vi "Project VIs.vi"(8 "Error In":errorcluster, 11 "Proejct Target App In":refnum<vi>) -> (0 "Error Out":errorcluster, 2 "VIs":T1[](array[typedef]), 3 "Project Target App Out":refnum<vi>)   [LabVIEW 2017, in "Bookmark Manager.lvlib"]
uses:
  Bookmark Manager.lvlib
  Controls/VI Information.ctl
  Controls/Application Information.ctl
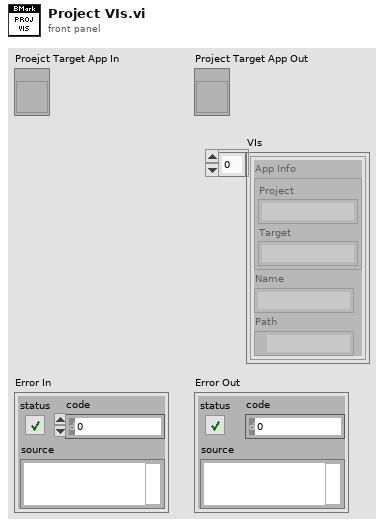
[diagram p1: front panel]
types:
  T1 = typedef "Bookmark Manager.lvlib/VI Information.ctl" = cluster{"App Info":T2, "Name":string, "Path":path}
  T2 = typedef "Bookmark Manager.lvlib/Application Information.ctl" = cluster{"Project":string, "Target":string}
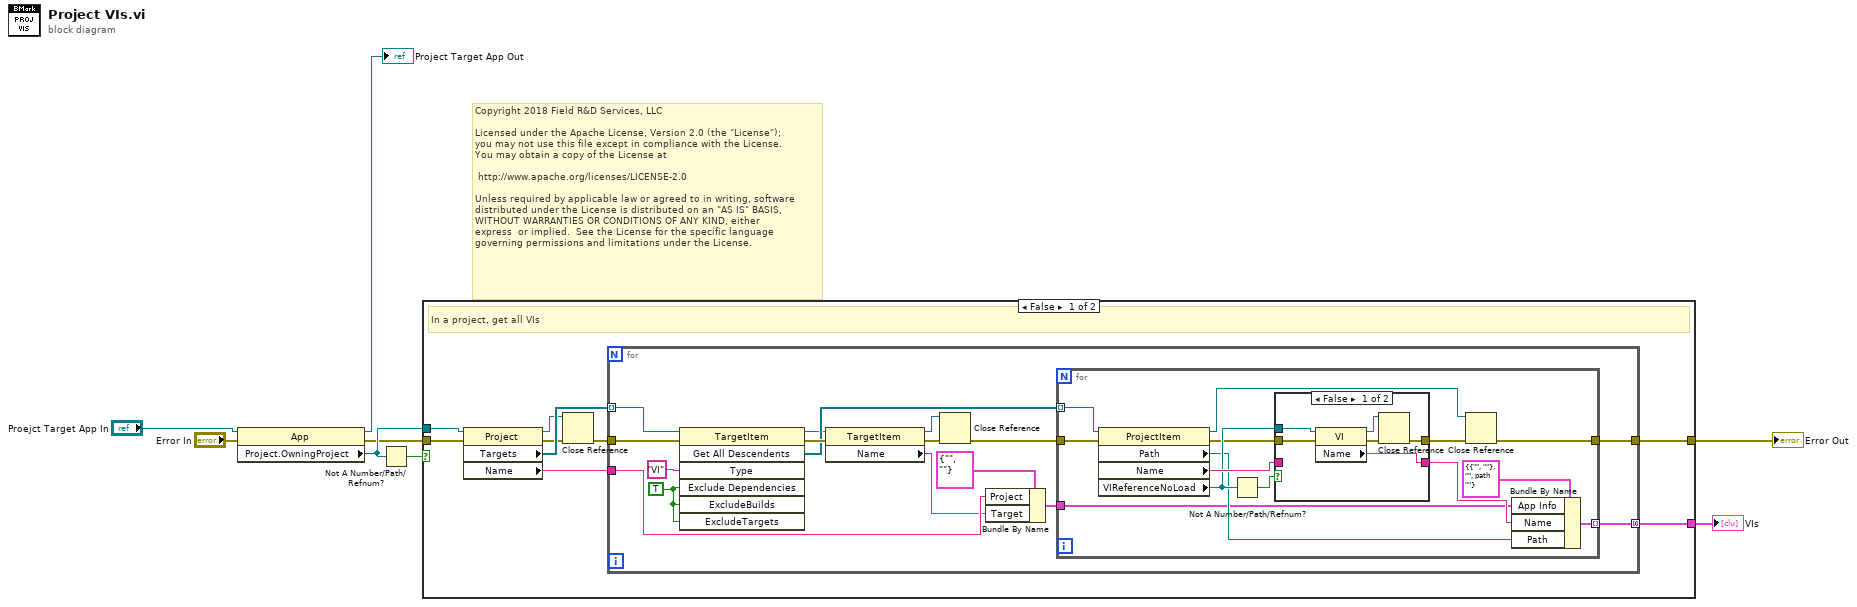
[diagram p0: block diagram]
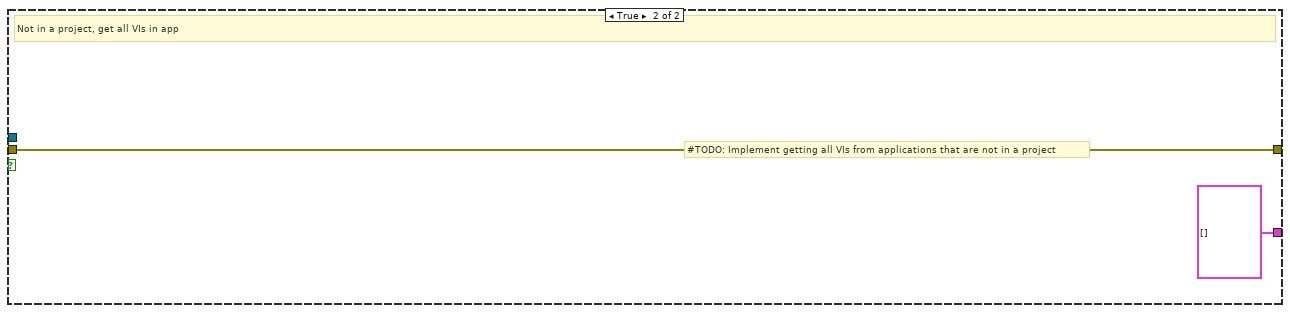
[diagram p3: hidden frame]
diagram:
  # "Copyright 2018 Field R&D Services, LLC\n\nLicensed under the Apache License, Version 2.0 (the \"License\");\nyou may not use this file except in compliance with the License.\nYou may obtain a copy of the License at\n\n\thttp://www.apache.org/licenses/LICENSE-2.0\n\nUnless required by applicable law or agreed to in writing, software\ndistributed under the License is distributed on an \"AS IS\" BASIS,\nWITHOUT WARRANTIES OR CONDITIONS OF ANY KIND, either \nexpress  or implied.  See the License for the specific language \ngoverning permissions and limitations under the License."
  n1 = property class="App"(reference="Proejct Target App In", error in="Error In") -> (reference out=→"Project Target App Out":refnum<vi>, error out=w3:errorcluster, "Project.OwningProject"=w7:refnum<vi>)
  n2 = Not A Number/Path/Refnum?(number/path/refnum=w7) -> (NaN/Path/Refnum?=w6:bool)
  n3 = case shown="False" w6 {
    tunnel: w7 -> [w16 _]
    tunnel: w3 -> [w17 w57]
    tunnel: [w12 w57] -> w8
    tunnel: [w9 T1[] []] -> w1
    frame False {
      # "In a project, get all VIs"
      n4 = property class="Project"(reference=w16, error in=w17) -> (reference out=w10:refnum<vi>, error out=w14:errorcluster, "Targets"=w15:refnum<vi>[], "Name"=w13:string)
      n5 = Close Reference(reference=w10, error in (no error)=w14) -> (error out=w11:errorcluster)
      n6 = for {
        tunnel: w15 -> [w33] mode=indexing
        tunnel: w11 -> [w32]
        tunnel: w13 -> [w24]
        tunnel: [w21] -> w9 mode=concatenating
        tunnel: [w20] -> w12
        w30 = TRUE ("ExcludeDependencies")
        n7 = invoke class="TargetItem" method="Get All Descendents"(reference=w33, error in=w32, "Type"="VI", "Exclude Dependencies"=w30, "ExcludeBuilds"=w30, "ExcludeTargets"=w30) -> (reference out=w27:refnum<vi>, error out=w29:errorcluster, "All Descendents"=w28:refnum<vi>[])  [unwired: 1 in, 4 out]
        n8 = property class="TargetItem"(reference=w27, error in=w29) -> (reference out=w18:refnum<vi>, error out=w26:errorcluster, "Name"=w23:string)
        n9 = Close Reference(reference=w18, error in (no error)=w26) -> (error out=w19:errorcluster)
        n10 = Bundle By Name(cluster=T2 {"Project"="", "Target"=""} ("App Info"), "Project"=w24, "Target"=w23) -> (w22:T2)
        n11 = for {
          tunnel: w19 -> [w47]
          tunnel: w28 -> [w46] mode=indexing
          tunnel: w22 -> [w36]
          tunnel: [w35] -> w21 mode=indexing
          tunnel: [w34] -> w20
          n12 = property class="ProjectItem"(reference=w46, error in=w47) -> (reference out=w41:refnum<vi>, error out=w42:errorcluster, "Path"=w37:path, "Name"=w44:string, "VIReferenceNoLoad"=w43:refnum<vi>)
          n13 = Not A Number/Path/Refnum?(number/path/refnum=w43) -> (NaN/Path/Refnum?=w45:bool)
          n14 = case shown="False" w45 {
            tunnel: w44 -> [_ w55]
            tunnel: [w48 w55] -> w38
            tunnel: w43 -> [w53 _]
            tunnel: w42 -> [w52 w54]
            tunnel: [w49 w54] -> w40
            frame False {
              n15 = property class="VI"(reference=w53, error in=w52) -> (reference out=w51:refnum<vi>, error out=w50:errorcluster, "Name"=w48:string)
              n16 = Close Reference(reference=w51, error in (no error)=w50) -> (error out=w49:errorcluster)
            }
            frame True {
            }
          }
          n17 = Close Reference(reference=w41, error in (no error)=w40) -> (error out=w34:errorcluster)
          n18 = Bundle By Name(cluster=T1 {"App Info"={"Project"="", "Target"=""}, "Name"="", "Path"=path ""} ("VI Info"), "App Info"=w36, "Name"=w38, "Path"=w37) -> (w35:T1)
        }
      }
    }
    frame True {
      # "#TODO: Implement getting all VIs from applications that are not in a project"
      # "Not in a project, get all VIs in app"
    }
  }
  "Error Out" <- w8
  "VIs" <- w1
